vi "Del.vi"(3 "User":string, 4 "Pass":string, 5 "Datos":string) -> (0 "Del OK?":bool, 1 "Usuario":string, 2 "Directorio Nuevo":string)   [LabVIEW 2017]
panel:
  out "Arreglo nuevo":string[][](array[string])
  out "Usuarios":string[][](array[string])
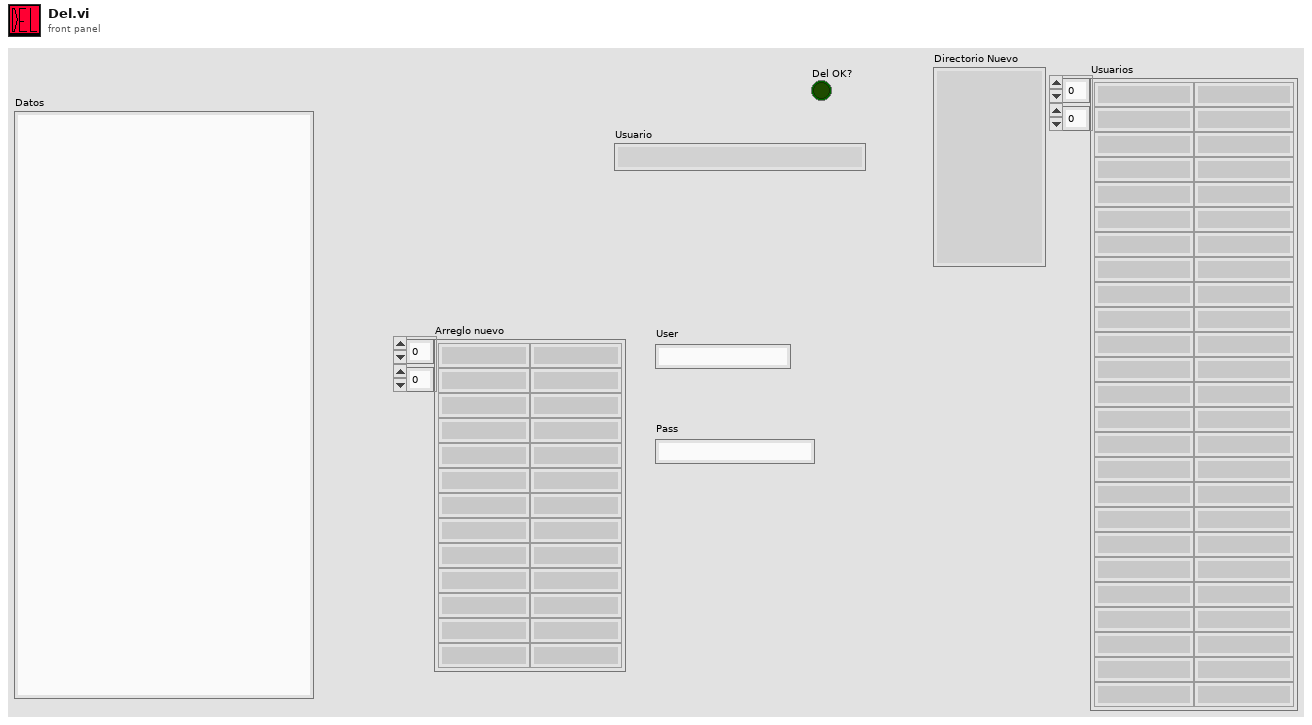
[diagram p1: front panel]
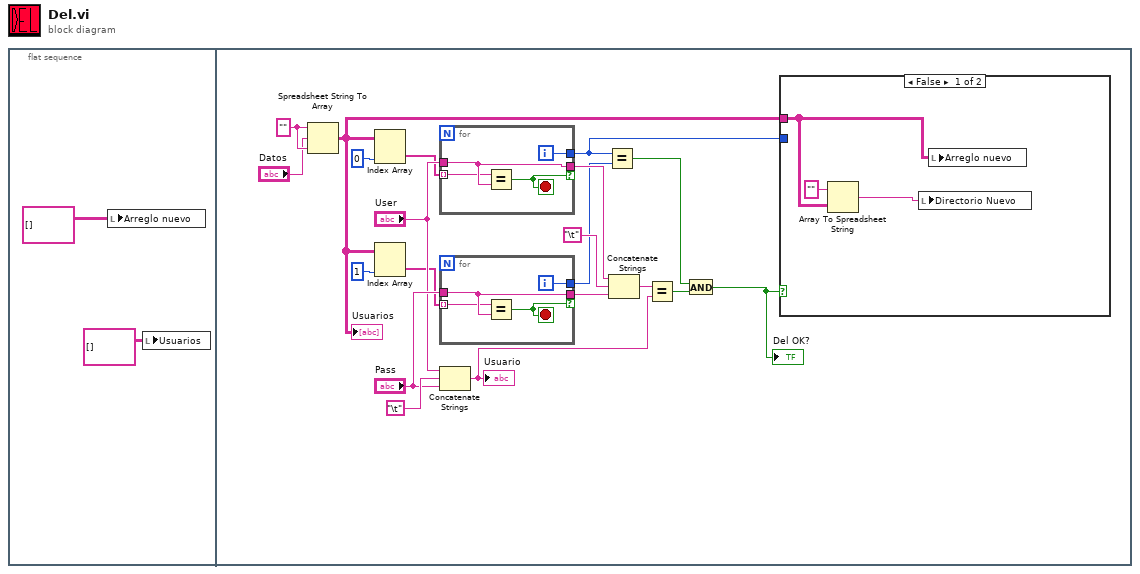
[diagram p0: block diagram]
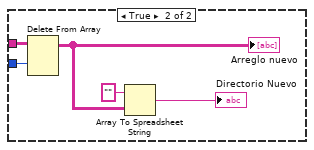
[diagram p2: hidden frame]
diagram:
  n1 = flat-sequence {
    frame #0 {
      n2 = local write "Arreglo nuevo"(string[][] [] ("array w/ subset deleted")) -> ()
      n3 = local write "Usuarios"(string[][] [] ("array")) -> ()
    }
    frame #1 {
      w21 = "" ("format string")
      n4 = Spreadsheet String To Array(format string=w21, spreadsheet string="Datos", array type (2D Dbl)=w21) -> (array=w5:string[][])  [unwired: 1 in]
      "Usuarios" <- w5
      n5 = Index Array(array=w5, index (col)=0 ("disabled index (col)")) -> (element=w7:string[])  [unwired: 1 in]
      n6 = Index Array(array=w5, index (col)=1 ("disabled index (col)")) -> (element=w6:string[])  [unwired: 1 in]
      n7 = for {
        tunnel: w7 -> [w35] mode=indexing
        tunnel: "User" -> [w38]
        tunnel: [w38] -> w18 if=w37
        tunnel: [w36] -> w4
        i -> [w36]
        stop <- w37 stop-if-true
        n8 = Equal?(x=w35, y=w38) -> (x = y?=w37:bool)
      }
      n9 = for {
        tunnel: w6 -> [w33] mode=indexing
        tunnel: "Pass" -> [w34]
        tunnel: [w34] -> w17 if=w31
        tunnel: [w32] -> w8
        i -> [w32]
        stop <- w31 stop-if-true
        n10 = Equal?(x=w33, y=w34) -> (x = y?=w31:bool)
      }
      n11 = Concatenate Strings("User", "\t", "Pass") -> (w14:string)
      "Usuario" <- w14
      n12 = Equal?(x=w4, y=w8) -> (x = y?=w9:bool)
      n13 = Concatenate Strings(w18, "\t", w17) -> (w15:string)
      n14 = Equal?(x=w15, y=w14) -> (x = y?=w10:bool)
      n15 = And(x=w9, y=w10) -> (x .and. y?=w3:bool)
      "Del OK?" <- w3
      n16 = case shown="False" w3 {
        tunnel: w5 -> [w24 w30]
        tunnel: w4 -> [_ w29]
        frame False {
          n17 = Array To Spreadsheet String(array=w24, 3:"" ("format string")) -> (spreadsheet string=w23:string)  [unwired: 1 in]
          n18 = local write "Directorio Nuevo"(w23) -> ()
          n19 = local write "Arreglo nuevo"(w24) -> ()
        }
        frame True {
          n20 = Delete From Array(array=w30, index (row)=w29) -> (array with subset deleted=w27:string[][])  [unwired: 2 in, 1 out]
          "Arreglo nuevo" <- w27
          n21 = Array To Spreadsheet String(array=w27, 3:"" ("format string")) -> (spreadsheet string=→"Directorio Nuevo":string)  [unwired: 1 in]
        }
      }
    }
  }
